vi "Create Events.vi"(0 "Display State In":T2={"Nspeakers"=13, "actions"=[], "Wspeaker"=13, "Wmic"=13, "sel mic"=13, "hover"={"type"=enum."None", "index"=0}, "locked"=FALSE, "states"=[], "sel speak"=13, "selected"=refnum, "Events"={"Mic change"=refnum, "Selection change"=refnum}}, 9 "Container State":T6, 11 "error in (no error)":errorcluster) -> (4 "Display State Out":T2={"Nspeakers"=13, "actions"=[], "Wspeaker"=13, "Wmic"=13, "sel mic"=13, "hover"={"type"=enum."None", "index"=0}, "locked"=FALSE, "states"=[], "sel speak"=13, "selected"=refnum, "Events"={"Mic change"=refnum, "Selection change"=refnum}}, 8 "Events":T1, 15 "error out":errorcluster)   [LabVIEW 2015, in "HRTF Config.xctl"]
uses:
  HRTF Config.xctl
  <vilib>/_xctls/Container State.ctl
  State.vi
  Hover Data.ctl
  Hover Item.ctl
  Speaker State.ctl
  Events.ctl
  Selection changed.ctl
  Mic change.ctl
  <vilib>/_xctls/XControlSupport.lvlib
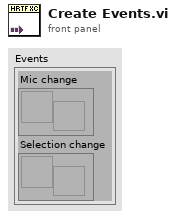
[diagram p1: front panel]
types:
  T1 = typedef "HRTF Config.xctl/Events.ctl" = cluster{"Mic change":refnum<user-event>, "Selection change":refnum<user-event>}
  T2 = typedef "HRTF Config.xctl/State.vi" = cluster{"Nspeakers":i32, "actions":string[], "Wspeaker":i32, "Wmic":i32, "sel mic":i32, "hover":T3, "locked":bool, "states":T5[], "sel speak":i32, "selected":refnum<vi>, "Events":T1}
  T3 = typedef "HRTF Config.xctl/Hover Data.ctl" = cluster{"type":T4, "index":i32}
  T4 = typedef "HRTF Config.xctl/Hover Item.ctl" = enum16{"None", "Speaker", "Mic"}
  T5 = typedef "HRTF Config.xctl/Speaker State.ctl" = cluster{"right cal":bool, "left cal":bool, "selected":bool}
  T6 = typedef "XControlSupport.lvlib/Container State.ctl" = cluster{"Indicator?":bool, "Run Mode?":bool, " Refnum":refnum<vi>}
  T7 = typedef "HRTF Config.xctl/Selection changed.ctl" = cluster{"Value":i32[]}
  T8 = typedef "HRTF Config.xctl/Mic change.ctl" = cluster{"Value":i32}
  T9 = cluster{"Event Data":refnum<user-event>, "Event Data":refnum<user-event>}
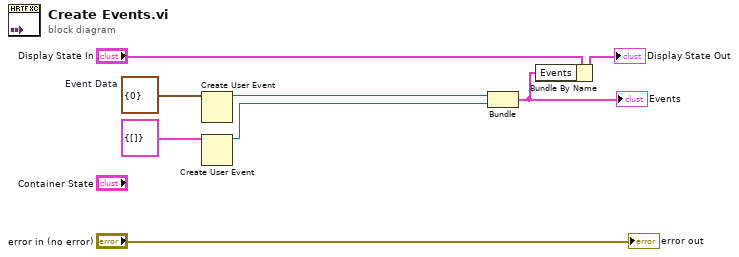
[diagram p0: block diagram]
diagram:
  w5 = T8 {"Value"=0}  # Event Data
  n1 = Create User Event(user event datatype=w5) -> (user event=w4:refnum<user-event>)  [unwired: 1 in, 1 out]
  n2 = Create User Event(user event datatype=T7 {"Value"=[]} ("Event Data")) -> (user event=w2:refnum<user-event>)  [unwired: 1 in, 1 out]
  n3 = Bundle("Event Data"=w4, "Event Data"=w2) -> (w1:T9)  [unwired: 1 in]
  "Events" <- w1
  n4 = Bundle By Name(cluster="Display State In", "Events"=w1) -> (→"Display State Out":T2)
  "error out" <- "error in (no error)"
